vi "Transcriptor LabVIEW to C code Translator 2.vi"(0 "Input":variant=variant("Function Name"=variant(string "Strip Path"), "Input Datatypes"=variant(string[] ["error", "int"]), "Inputs"=variant(string[] ["error in", "x"]), "Node refnum"=variant(refnum<vi> refnum), "Output Datatypes"=variant(string[] ["int"]), "Outputs"=variant(string[] ["a"])), 11 "error in (no error)":errorcluster) -> (4 "Output":variant=variant("Defines"=variant(string[] []), "Includes"=variant(string[] []), "Replaced Code"=variant(string "/* LabVIEW system function 'Strip Path' not found. */")), 15 "error out":errorcluster)   [LabVIEW 2014]
doc: "An example of how to create the Translator to convert the LabVIEW VIs to Arduino C code."
panel:
  out "Outputs":string[](array[string])
  out "Inputs":string[](array[string])
  out "Output Datatypes":string[](array[string])
  out "Input Datatypes":string[](array[string])
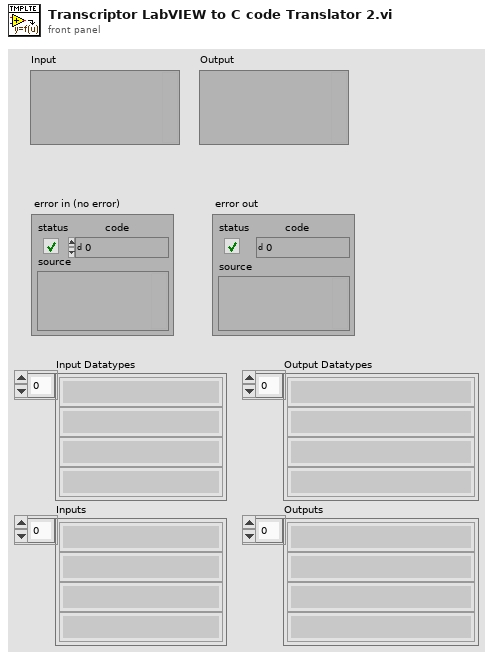
[diagram p1: front panel]
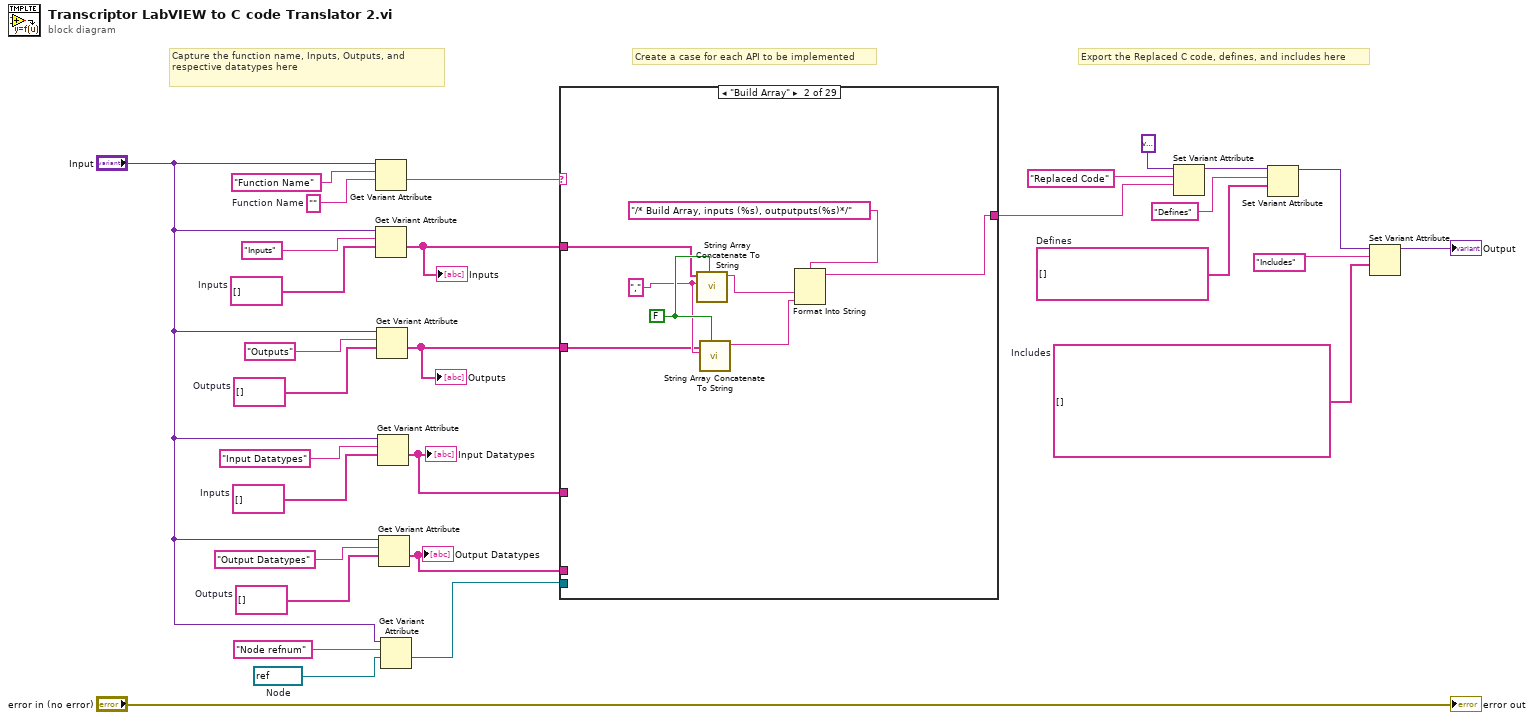
[diagram p0: block diagram]
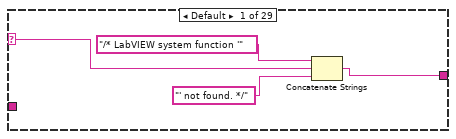
[diagram p2: hidden frame]
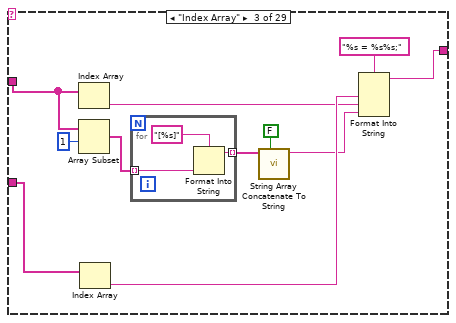
[diagram p3: hidden frame]
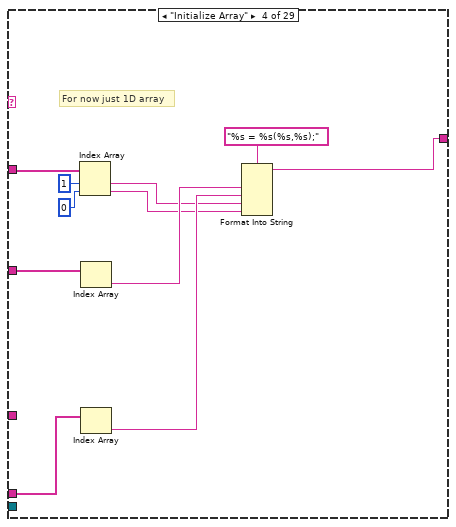
[diagram p4: hidden frame]
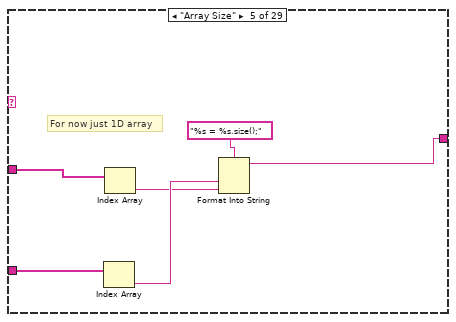
[diagram p5: hidden frame]
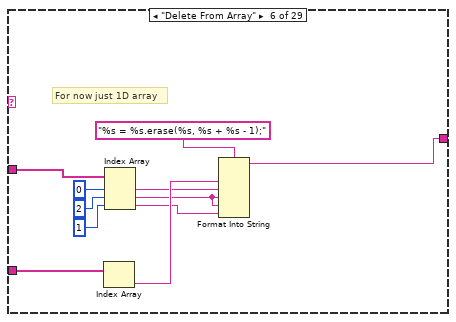
[diagram p6: hidden frame]
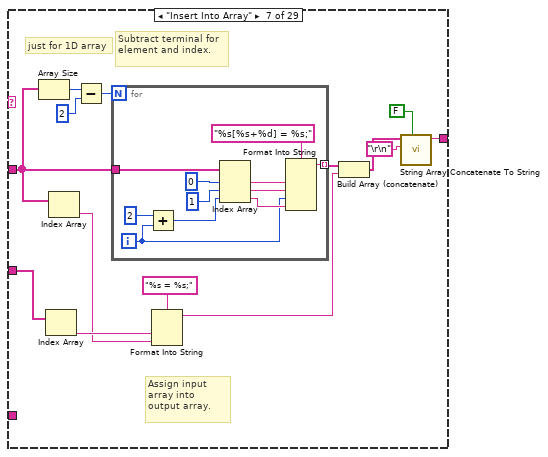
[diagram p7: hidden frame]
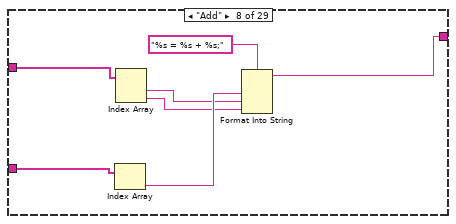
[diagram p8: hidden frame]
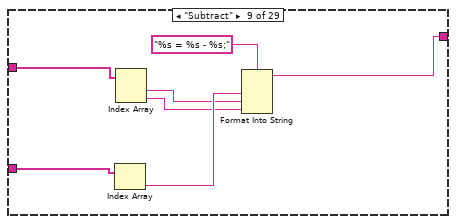
[diagram p9: hidden frame]
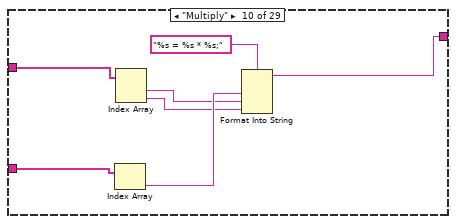
[diagram p10: hidden frame]
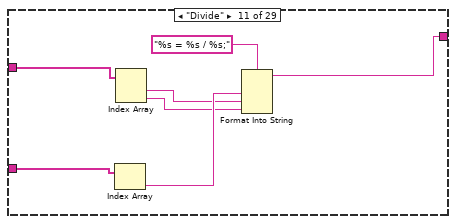
[diagram p11: hidden frame]
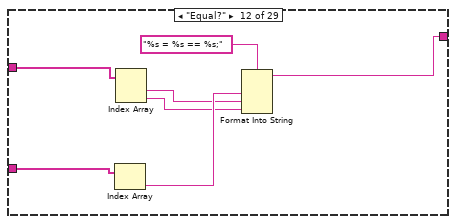
[diagram p12: hidden frame]
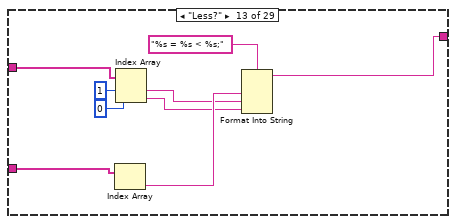
[diagram p13: hidden frame]
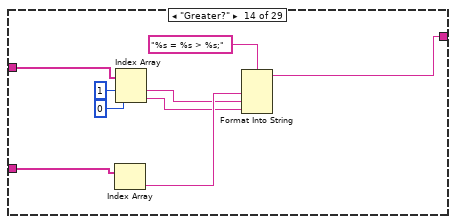
[diagram p14: hidden frame]
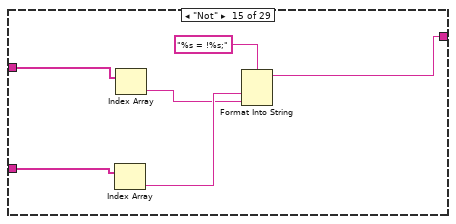
[diagram p15: hidden frame]
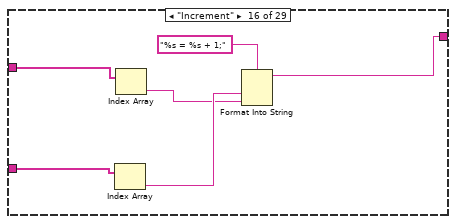
[diagram p16: hidden frame]
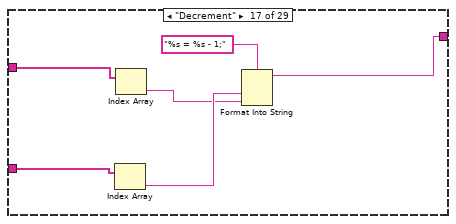
[diagram p17: hidden frame]
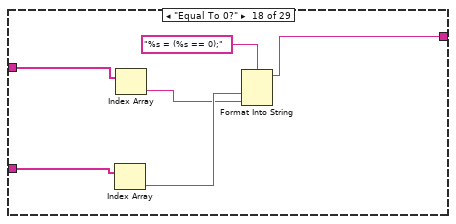
[diagram p18: hidden frame]
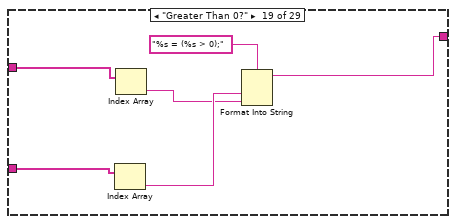
[diagram p19: hidden frame]
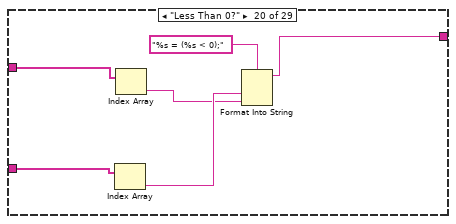
[diagram p20: hidden frame]
diagram:
  w3 = refnum<vi> refnum  # Node
  w7 = string[] []  # Defines
  w15 = string[] []  # Outputs
  w16 = string[] []  # Inputs
  w21 = string[] []  # Includes
  w26 = string[] []  # Outputs
  w27 = string[] []  # Inputs
  w28 = ""  # Function Name
  # "Capture the function name, Inputs, Outputs, and respective datatypes here"
  # "Export the Replaced C code, defines, and includes here"
  # "Create a case for each API to be implemented"
  n1 = Get Variant Attribute(Variant="Input", name="Function Name", default value (empty Variant)=w28) -> (value=w23:string)  [unwired: 1 in, 3 out]
  n2 = Get Variant Attribute(Variant="Input", name="Inputs", default value (empty Variant)=w27) -> (value=w12:string[])  [unwired: 1 in, 3 out]
  "Inputs" <- w12
  n3 = Get Variant Attribute(Variant="Input", name="Outputs", default value (empty Variant)=w26) -> (value=w13:string[])  [unwired: 1 in, 3 out]
  "Outputs" <- w13
  n4 = Get Variant Attribute(Variant="Input", name="Input Datatypes", default value (empty Variant)=w16) -> (value=w6:string[])  [unwired: 1 in, 3 out]
  "Input Datatypes" <- w6
  n5 = Get Variant Attribute(Variant="Input", name="Output Datatypes", default value (empty Variant)=w15) -> (value=w1:string[])  [unwired: 1 in, 3 out]
  "Output Datatypes" <- w1
  n6 = Get Variant Attribute(Variant="Input", name="Node refnum", default value (empty Variant)=w3) -> (value=w2:refnum<vi>)  [unwired: 1 in, 3 out]
  n7 = case shown="\"Build Array\"" w23 {
    selector: w23 -> [w33 _ _ _ _ _ _ _ _ _ _ _ _ _ _ _ _ _ _ _ _ _ _ _ _ _ _ _ _]
    tunnel: [w31 w35 w49 w57 w68 w79 w96 w110 w117 w124 w131 w138 w147 w156 w163 w169 w175 w181 w187 w193 w199 w205 w211 w218 w225 w232 w238 w245 w252] -> w22
    tunnel: w12 -> [_ w39 w48 w67 w73 w84 w89 w116 w123 w130 w137 w144 w153 w162 w168 w174 w180 w186 w192 w198 w204 w210 w217 w224 w231 w237 w244 w251 w258]
    tunnel: w13 -> [_ w38 w53 w66 w71 w82 w92 w114 w121 w128 w135 w142 w151 w160 w166 w172 w178 w184 w190 w196 w202 w208 w215 w222 w229 w235 w242 w249 w256]
    tunnel: w6 -> [_ _ _ _ _ _ _ _ _ _ _ _ _ _ _ _ _ _ _ _ _ _ _ _ _ _ _ _ _]
    tunnel: w2 -> [_ _ _ _ _ _ _ _ _ _ _ _ _ _ _ _ _ _ _ _ _ _ _ _ _ _ _ _ _]
    tunnel: w1 -> [_ _ _ w62 _ _ _ _ _ _ _ _ _ _ _ _ _ _ _ _ _ _ _ _ _ _ _ _ _]
    frame Default {
      n8 = Concatenate Strings("/* LabVIEW system function '", w33, "' not found. */") -> (w31:string)
    }
    frame "Build Array" {
      w40 = "," ("string")
      w41 = FALSE ("insert last delimiter?")
      n9 = call "String Array Concatenate To String.vi"("insert last delimiter?"=w41, "Delimiter char"=w40, "Array String In"=w39) -> ("String"=w37:string)  [unwired: 8 in]
      n10 = call "String Array Concatenate To String.vi"("insert last delimiter?"=w41, "Delimiter char"=w40, "Array String In"=w38) -> ("String"=w36:string)  [unwired: 8 in]
      n11 = Format Into String(format string="/* Build Array, inputs (%s), outputputs(%s)*/" ("name"), w37, w36) -> (resulting string=w35:string)  [unwired: 2 in, 1 out]
    }
    frame "Index Array" {
      n12 = Index Array(array=w48) -> (element=w50:string)  [unwired: 1 in]
      n13 = Array Subset(array=w48, index=1) -> (w46:string[])  [unwired: 1 in]
      n14 = Index Array(array=w53) -> (element=w51:string)  [unwired: 1 in]
      n15 = for {
        tunnel: w46 -> [w55] mode=indexing
        tunnel: [w54] -> w44 mode=indexing
        n16 = Format Into String(format string="[%s]", w55) -> (resulting string=w54:string)  [unwired: 2 in, 1 out]
      }
      n17 = call "String Array Concatenate To String.vi"("insert last delimiter?"=FALSE, "Array String In"=w44) -> ("String"=w43:string)  [unwired: 9 in]
      n18 = Format Into String(format string="%s = %s%s;", w51, w50, w43) -> (resulting string=w49:string)  [unwired: 2 in, 1 out]
    }
    frame "Initialize Array" {
      # "For now just 1D array"
      n19 = Index Array(array=w67, index #1=1 ("index"), index #2=0 ("index")) -> (element #1=w59:string, element #2=w58:string)
      n20 = Index Array(array=w66) -> (element=w64:string)  [unwired: 1 in]
      n21 = Index Array(array=w62) -> (element=w63:string)  [unwired: 1 in]
      n22 = Format Into String(format string="%s = %s(%s,%s);", w64, w63, w59, w58) -> (resulting string=w57:string)  [unwired: 2 in, 1 out]
    }
    frame "Array Size" {
      # "For now just 1D array"
      n23 = Index Array(array=w71) -> (element=w70:string)  [unwired: 1 in]
      n24 = Index Array(array=w73) -> (element=w69:string)  [unwired: 1 in]
      n25 = Format Into String(format string="%s = %s.size();", w70, w69) -> (resulting string=w68:string)  [unwired: 2 in, 1 out]
    }
    frame "Delete From Array" {
      # "For now just 1D array"
      n26 = Index Array(array=w82) -> (element=w81:string)  [unwired: 1 in]
      n27 = Index Array(array=w84, index #1=0 ("index"), index #2=2 ("index"), index #3=1 ("index")) -> (element #1=w80:string, element #2=w75:string, element #3=w74:string)
      n28 = Format Into String(format string="%s = %s.erase(%s, %s + %s - 1);", w81, w80, w75, w75, w74) -> (resulting string=w79:string)  [unwired: 2 in, 1 out]
    }
    frame "Insert Into Array" {
      # "just for 1D array"
      # "Subtract terminal for element and index."
      # "Assign input array into output array."
      n29 = Array Size(array=w89) -> (size(s)=w94:i32)
      n30 = Index Array(array=w92) -> (element=w90:string)  [unwired: 1 in]
      n31 = Index Array(array=w89) -> (element=w88:string)  [unwired: 1 in]
      n32 = Subtract(x=w94, y=2) -> (x-y=w95:i32)
      n33 = for {
        N: w95 -> [_]
        tunnel: w89 -> [w106]
        tunnel: [w107] -> w87 mode=indexing
        i -> [w102]
        n34 = Add(x=2, y=w102) -> (x+y=w101:i32)
        n35 = Index Array(array=w106, index #1=0 ("index"), index #2=1 ("index"), index #3=w101) -> (element #1=w99:string, element #2=w108:string, element #3=w104:string)
        n36 = Format Into String(format string="%s[%s+%d] = %s;", w99, w108, w102, w104) -> (resulting string=w107:string)  [unwired: 2 in, 1 out]
      }
      n37 = Format Into String(format string="%s = %s;", w90, w88) -> (resulting string=w86:string)  [unwired: 2 in, 1 out]
      n38 = Build Array (concatenate)(w87, w86) -> (w85:string[])
      n39 = call "String Array Concatenate To String.vi"("insert last delimiter?"=FALSE, "Delimiter char"="\r\n", "Array String In"=w85) -> ("String"=w96:string)  [unwired: 8 in]
    }
    frame "Add" {
      n40 = Index Array(array=w114) -> (element=w113:string)  [unwired: 1 in]
      n41 = Index Array(array=w116) -> (element #1=w112:string, element #2=w111:string)  [unwired: 2 in]
      n42 = Format Into String(format string="%s = %s + %s;", w113, w112, w111) -> (resulting string=w110:string)  [unwired: 2 in, 1 out]
    }
    frame "Subtract" {
      n43 = Index Array(array=w121) -> (element=w120:string)  [unwired: 1 in]
      n44 = Index Array(array=w123) -> (element #1=w119:string, element #2=w118:string)  [unwired: 2 in]
      n45 = Format Into String(format string="%s = %s - %s;", w120, w119, w118) -> (resulting string=w117:string)  [unwired: 2 in, 1 out]
    }
    frame "Multiply" {
      n46 = Index Array(array=w128) -> (element=w127:string)  [unwired: 1 in]
      n47 = Index Array(array=w130) -> (element #1=w126:string, element #2=w125:string)  [unwired: 2 in]
      n48 = Format Into String(format string="%s = %s * %s;", w127, w126, w125) -> (resulting string=w124:string)  [unwired: 2 in, 1 out]
    }
    frame "Divide" {
      n49 = Index Array(array=w135) -> (element=w134:string)  [unwired: 1 in]
      n50 = Index Array(array=w137) -> (element #1=w133:string, element #2=w132:string)  [unwired: 2 in]
      n51 = Format Into String(format string="%s = %s / %s;", w134, w133, w132) -> (resulting string=w131:string)  [unwired: 2 in, 1 out]
    }
    frame "Equal?" {
      n52 = Index Array(array=w142) -> (element=w141:string)  [unwired: 1 in]
      n53 = Index Array(array=w144) -> (element #1=w140:string, element #2=w139:string)  [unwired: 2 in]
      n54 = Format Into String(format string="%s = %s == %s;", w141, w140, w139) -> (resulting string=w138:string)  [unwired: 2 in, 1 out]
    }
    frame "Less?" {
      n55 = Index Array(array=w151) -> (element=w150:string)  [unwired: 1 in]
      n56 = Index Array(array=w153, index #1=1 ("index"), index #2=0 ("index")) -> (element #1=w149:string, element #2=w148:string)
      n57 = Format Into String(format string="%s = %s < %s;", w150, w149, w148) -> (resulting string=w147:string)  [unwired: 2 in, 1 out]
    }
    frame "Greater?" {
      n58 = Index Array(array=w160) -> (element=w159:string)  [unwired: 1 in]
      n59 = Index Array(array=w162, index #1=1 ("index"), index #2=0 ("index")) -> (element #1=w158:string, element #2=w157:string)
      n60 = Format Into String(format string="%s = %s > %s;", w159, w158, w157) -> (resulting string=w156:string)  [unwired: 2 in, 1 out]
    }
    frame "Not" {
      n61 = Index Array(array=w166) -> (element=w165:string)  [unwired: 1 in]
      n62 = Index Array(array=w168) -> (element=w164:string)  [unwired: 1 in]
      n63 = Format Into String(format string="%s = !%s;", w165, w164) -> (resulting string=w163:string)  [unwired: 2 in, 1 out]
    }
    frame "Increment" {
      n64 = Index Array(array=w172) -> (element=w171:string)  [unwired: 1 in]
      n65 = Index Array(array=w174) -> (element=w170:string)  [unwired: 1 in]
      n66 = Format Into String(format string="%s = %s + 1;", w171, w170) -> (resulting string=w169:string)  [unwired: 2 in, 1 out]
    }
    frame "Decrement" {
      n67 = Index Array(array=w178) -> (element=w177:string)  [unwired: 1 in]
      n68 = Index Array(array=w180) -> (element=w176:string)  [unwired: 1 in]
      n69 = Format Into String(format string="%s = %s - 1;", w177, w176) -> (resulting string=w175:string)  [unwired: 2 in, 1 out]
    }
    frame "Equal To 0?" {
      n70 = Index Array(array=w184) -> (element=w183:string)  [unwired: 1 in]
      n71 = Index Array(array=w186) -> (element=w182:string)  [unwired: 1 in]
      n72 = Format Into String(format string="%s = (%s == 0);", w183, w182) -> (resulting string=w181:string)  [unwired: 2 in, 1 out]
    }
    frame "Greater Than 0?" {
      n73 = Index Array(array=w190) -> (element=w189:string)  [unwired: 1 in]
      n74 = Index Array(array=w192) -> (element=w188:string)  [unwired: 1 in]
      n75 = Format Into String(format string="%s = (%s > 0);", w189, w188) -> (resulting string=w187:string)  [unwired: 2 in, 1 out]
    }
    frame "Less Than 0?" {
      n76 = Index Array(array=w196) -> (element=w195:string)  [unwired: 1 in]
      n77 = Index Array(array=w198) -> (element=w194:string)  [unwired: 1 in]
      n78 = Format Into String(format string="%s = (%s < 0);", w195, w194) -> (resulting string=w193:string)  [unwired: 2 in, 1 out]
    }
    frame "Greater Or Equal To 0?" {
      n79 = Index Array(array=w202) -> (element=w201:string)  [unwired: 1 in]
      n80 = Index Array(array=w204) -> (element=w200:string)  [unwired: 1 in]
      n81 = Format Into String(format string="%s = (%s >= 0);", w201, w200) -> (resulting string=w199:string)  [unwired: 2 in, 1 out]
    }
    frame "Less Or Equal To 0?" {
      n82 = Index Array(array=w208) -> (element=w207:string)  [unwired: 1 in]
      n83 = Index Array(array=w210) -> (element=w206:string)  [unwired: 1 in]
      n84 = Format Into String(format string="%s = (%s <= 0);", w207, w206) -> (resulting string=w205:string)  [unwired: 2 in, 1 out]
    }
    frame "Greater Or Equal?" {
      n85 = Index Array(array=w215) -> (element=w214:string)  [unwired: 1 in]
      n86 = Index Array(array=w217) -> (element #1=w213:string, element #2=w212:string)  [unwired: 2 in]
      n87 = Format Into String(format string="%s = (%s >= %s);", w214, w213, w212) -> (resulting string=w211:string)  [unwired: 2 in, 1 out]
    }
    frame "Less Or Equal?" {
      n88 = Index Array(array=w222) -> (element=w221:string)  [unwired: 1 in]
      n89 = Index Array(array=w224) -> (element #1=w220:string, element #2=w219:string)  [unwired: 2 in]
      n90 = Format Into String(format string="%s = (%s <= %s);", w221, w220, w219) -> (resulting string=w218:string)  [unwired: 2 in, 1 out]
    }
    frame "Not Equal?" {
      n91 = Index Array(array=w229) -> (element=w228:string)  [unwired: 1 in]
      n92 = Index Array(array=w231) -> (element #1=w227:string, element #2=w226:string)  [unwired: 2 in]
      n93 = Format Into String(format string="%s = (%s != %s);", w228, w227, w226) -> (resulting string=w225:string)  [unwired: 2 in, 1 out]
    }
    frame "Not Equal To 0?" {
      n94 = Index Array(array=w235) -> (element=w234:string)  [unwired: 1 in]
      n95 = Index Array(array=w237) -> (element=w233:string)  [unwired: 1 in]
      n96 = Format Into String(format string="%s = (%s != 0);", w234, w233) -> (resulting string=w232:string)  [unwired: 2 in, 1 out]
    }
    frame "And" {
      n97 = Index Array(array=w242) -> (element=w241:string)  [unwired: 1 in]
      n98 = Index Array(array=w244) -> (element #1=w240:string, element #2=w239:string)  [unwired: 2 in]
      n99 = Format Into String(format string="%s = %s AND %s;", w241, w240, w239) -> (resulting string=w238:string)  [unwired: 2 in, 1 out]
    }
    frame "Or" {
      n100 = Index Array(array=w249) -> (element=w248:string)  [unwired: 1 in]
      n101 = Index Array(array=w251) -> (element #1=w247:string, element #2=w246:string)  [unwired: 2 in]
      n102 = Format Into String(format string="%s = %s OR %s;", w248, w247, w246) -> (resulting string=w245:string)  [unwired: 2 in, 1 out]
    }
    frame "Exclusive Or" {
      n103 = Index Array(array=w256) -> (element=w255:string)  [unwired: 1 in]
      n104 = Index Array(array=w258) -> (element #1=w254:string, element #2=w253:string)  [unwired: 2 in]
      n105 = Format Into String(format string="%s = %s XOR %s;", w255, w254, w253) -> (resulting string=w252:string)  [unwired: 2 in, 1 out]
    }
  }
  n106 = Set Variant Attribute(Variant=variant ("variant"), name="Replaced Code", value=w22) -> (Variant out=w10:variant)  [unwired: 1 in, 2 out]
  n107 = Set Variant Attribute(Variant=w10, name="Defines", value=w7) -> (Variant out=w9:variant)  [unwired: 1 in, 2 out]
  n108 = Set Variant Attribute(Variant=w9, name="Includes", value=w21) -> (Variant out=→"Output":variant)  [unwired: 1 in, 2 out]
  "error out" <- "error in (no error)"
